vi "Auto Transmission and Manual control.vi"(0 "Drive":T4, 1 "Force which gear it is in":bool, 3 "Forced high gear?":bool, 5 "Commanded speeds":cluster{"Steer":dbl, "Throttle":dbl}, 9 "from Shift":T1, 11 "error in (no error)":errorcluster, 12 "All Shifter Constants":T2) -> (4 "Drive out":T4, 6 "in High Gear?":bool, 8 "Robot speed in FPS":dbl, 10 "To shift":T1, 14 "Recomended Gear (may be in that gear)":bool, 15 "error out":errorcluster)   [LabVIEW 2013]
uses:
  Drive typedef.ctl
  Drive Motors Typedef.ctl
  GearBox Typedef.ctl
  <vilib>/Rock Robotics/WPI/MotorControl/WPI_MotorControlDeviceRef.ctl
  <vilib>/Rock Robotics/SystemInterfaces/Typedef/FPGA_TypedefDigitalModule.ctl
  <vilib>/Rock Robotics/SystemInterfaces/DIO/FPGA_DIOPWMChannel.ctl
  <vilib>/Rock Robotics/WPI/PWM/WPI_PWMDeadband.ctl
  <vilib>/Rock Robotics/WPI/CAN/Jaguar/SubVIs/WPI_CANJaguar_ControlMode.ctl
  <vilib>/Rock Robotics/WPI/PWM/WPI_PWMTransform_ConPane.ctl
  <vilib>/Rock Robotics/WPI/Solenoid/WPI_SolenoidDevRef.ctl
  <vilib>/Rock Robotics/SystemInterfaces/Typedef/FPGA_TypedefSolenoidModule.ctl
  <vilib>/Rock Robotics/WPI/Solenoid/WPI_SolenoidChannel.ctl
  Drive Sensor Typedef.ctl
  <vilib>/Rock Robotics/WPI/Encoder/WPI_EncoderDevRef.ctl
  <vilib>/Rock Robotics/SystemInterfaces/Encoder/FPGA_EncoderIdx.ctl
  <vilib>/Rock Robotics/SystemInterfaces/Counter/FPGA_CounterCtrSystemIndex.ctl
  <vilib>/Rock Robotics/WPI/Encoder/WPI_EncoderType.ctl
  <vilib>/Rock Robotics/WPI/Gyro/WPI_GyroDevRef.ctl
  <vilib>/Rock Robotics/SystemInterfaces/Typedef/FPGA_TypedefAnalogModule.ctl
  <vilib>/Rock Robotics/SystemInterfaces/AI/FPGA_AIChannel.ctl
  All Shifter Constants.ctl
  Shift Constants.ctl
  Shifter shift typedef.ctl
  <vilib>/Rock Robotics/WPI/Solenoid/WPI_SolenoidValue.ctl
  <vilib>/Rock Robotics/WPI/Solenoid/Deprecated/WPI_SolenoidGetBool.vi
  <vilib>/Rock Robotics/WPI/Solenoid/WPI_SolenoidSetEnum.vi
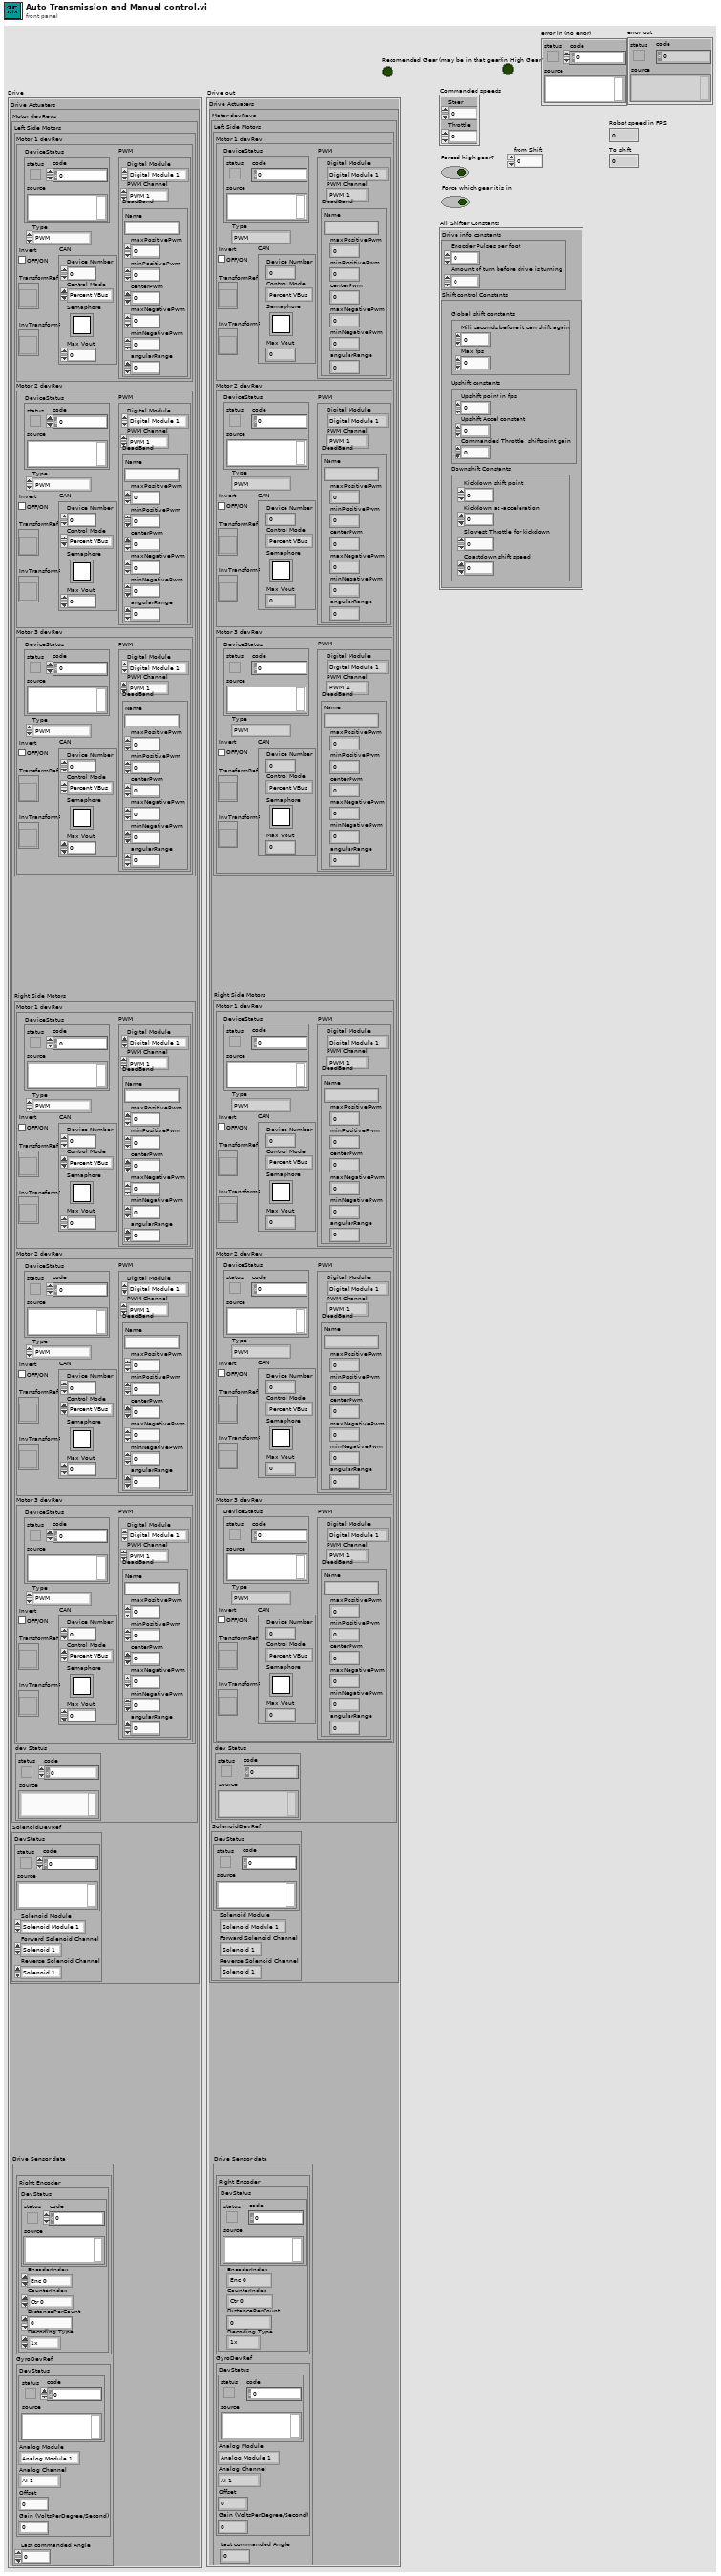
[diagram p1: front panel]
types:
  T1 = typedef "Shifter shift typedef.ctl" = u32
  T2 = typedef "All Shifter Constants.ctl" = cluster{"Drive info constants":cluster{"Enocder Pulses per foot":dbl, "Amount of turn before drive is turning":dbl}, "Shift control Constants":T3}
  T3 = typedef "Shift Constants.ctl" = cluster{"Global shift constants":cluster{"Mili seconds before it can shift again":u32, "Max fps":dbl}, "Upshift constants":cluster{"Upshift point in fps":dbl, "Upshift Accel constant":dbl, "Commanded Throttle  shiftpoint gain":dbl}, "Downshift Constants":cluster{"Kickdown shift point":dbl, "Kickdown at -acceleration":dbl, "Slowest Throttle for kickdown":dbl, "Coastdown shift speed":dbl}}
  T4 = typedef "Drive typedef.ctl" = cluster{"Drive Actuaters":cluster{"Motor devRevs":T5, "SolenoidDevRef":T14}, "Drive Sensor data":T17}
  T5 = typedef "Drive Motors Typedef.ctl" = cluster{"Left Side Motors":T6, "Right Side Motors":T6, "dev Status":errorcluster}
  T6 = typedef "GearBox Typedef.ctl" = cluster{"Motor 1 devRev":T7, "Motor 2 devRev":T7, "Motor 3 devRev":T7}
  T7 = typedef "WPI_MotorControlDeviceRef.ctl" = cluster{"DeviceStatus":errorcluster, "Type":enum16{"PWM", "CAN"}, "PWM":cluster{"Digital Module":T8, "PWM Channel":T9, "DeadBand":T10}, "CAN":cluster{"Device Number":u8, "Control Mode":T11, "Semaphore":T12, "Max Vout":dbl}, "Invert":bool, "TransformRef":T13, "InvTransformRef":T13}
  T8 = typedef "FPGA_TypedefDigitalModule.ctl" = enum16{"Digital Module 1", "Digital Module 2"}
  T9 = typedef "FPGA_DIOPWMChannel.ctl" = enum8{"PWM 1", "PWM 2", "PWM 3", "PWM 4", "PWM 5", "PWM 6", "PWM 7", "PWM 8", "PWM 9", "PWM 10", "Invalid"}
  T10 = typedef "WPI_PWMDeadband.ctl" = cluster{"Name":string, "maxPositivePwm":i32, "minPositivePwm":i32, "centerPwm":i32, "maxNegativePwm":i32, "minNegativePwm":i32, "angularRange":u16}
  T11 = typedef "WPI_CANJaguar_ControlMode.ctl" = enum8{"Percent VBus", "Current", "Speed", "Position", "Voltage"}
  T12 = typedef "Semaphore RefNum" = refnum<k1>
  T13 = typedef "WPI_PWMTransform_ConPane.ctl" = refnum<vi>
  T14 = typedef "WPI_SolenoidDevRef.ctl" = cluster{"DevStatus":errorcluster, "Solenoid Module":T15, "Forward Solenoid Channel":T16, "Reverse Solenoid Channel":T16}
  T15 = typedef "FPGA_TypedefSolenoidModule.ctl" = enum16{"Solenoid Module 1", "Solenoid Module 2"}
  T16 = typedef "WPI_SolenoidChannel.ctl" = enum8{"Solenoid 1", "Solenoid 2", "Solenoid 3", "Solenoid 4", "Solenoid 5", "Solenoid 6", "Solenoid 7", "Solenoid 8", "Invalid"}
  T17 = typedef "Drive Sensor Typedef.ctl" = cluster{"Encoders":cluster{"Right Encoder":T18}, "GyroDevRef":T22, "Last commanded Angle":dbl}
  T18 = typedef "WPI_EncoderDevRef.ctl" = cluster{"DevStatus":errorcluster, "EncoderIndex":T19, "CounterIndex":T20, "DistancePerCount":dbl, "Decoding Type":T21}
  T19 = typedef "FPGA_EncoderIdx.ctl" = enum8{"Enc 0", "Enc 1", "Enc 2", "Enc 3", "Invalid"}
  T20 = typedef "FPGA_CounterCtrSystemIndex.ctl" = enum8{"Ctr 0", "Ctr 1", "Ctr 2", "Ctr 3", "Ctr 4", "Ctr 5", "Ctr 6", "Ctr 7", "Invalid"}
  T21 = typedef "WPI_EncoderType.ctl" = enum16{"1x", "2x", "4x"}
  T22 = typedef "WPI_GyroDevRef.ctl" = cluster{"DevStatus":errorcluster, "Analog Module":T23, "Analog Channel":T24, "Offset":dbl, "Gain (VoltsPerDegree/Second)":dbl}
  T23 = typedef "FPGA_TypedefAnalogModule.ctl" = enum16{"Analog Module 1", "Analog Module 2"}
  T24 = typedef "FPGA_AIChannel.ctl" = enum8{"AI 1", "AI 2", "AI 3", "AI 4", "AI 5", "AI 6", "AI 7", "AI 8", "Invalid"}
  T25 = typedef "WPI_SolenoidValue.ctl" = enum16{"Off", "On", "Forward", "Reverse"}
  T26 = cluster{"Enocder Pulses per foot":dbl, "Amount of turn before drive is turning":dbl}
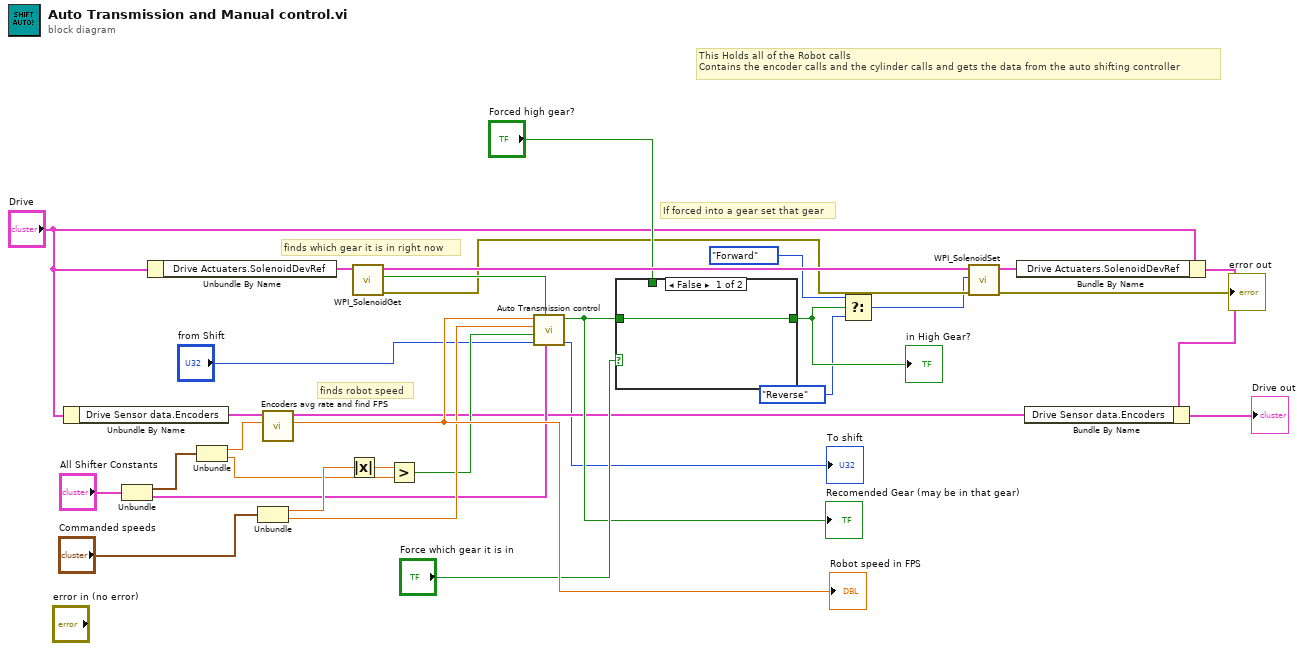
[diagram p0: block diagram]
diagram:
  # "finds which gear it is in right now"
  # "finds robot speed"
  # "If forced into a gear set that gear"
  # "This Holds all of the Robot calls\nContains the encoder calls and the cylinder calls and gets the data from the auto shifting controller"
  n1 = Unbundle By Name("Drive") -> ("Drive Sensor data.Encoders"=w31:cluster{"Right Encoder":T18})
  n2 = Unbundle("All Shifter Constants") -> ("Drive info constants"=w17:T26, "Shift control Constants"=w14:T3)
  n3 = Unbundle By Name("Drive") -> ("Drive Actuaters.SolenoidDevRef"=w29:T14)
  n4 = Unbundle(w17) -> ("Enocder Pulses per foot"=w16:dbl, "Amount of turn before drive is turning"=w15:dbl)
  n5 = Unbundle("Commanded speeds") -> ("Steer"=w25:dbl, "Throttle"=w26:dbl)
  n6 = call "Encoders avg rate and find FPS.vi"("encoder clicks per foot"=w16, "Encoders"=w31) -> ("Robot speed in FPS"=w30:dbl, "Encoders out"=w9:cluster{"Right Encoder":T18})  [unwired: 6 in, 2 out]
  "Robot speed in FPS" <- w30
  n7 = Absolute Value(x=w25) -> (abs(x)=w24:dbl)
  n8 = call-poly <vilib>:"WPI_SolenoidGet.vi"("SolenoidDevRef"=w29) -> ("error out"=w6:errorcluster, "Value"=w28:bool, "SolenoidDevRef"=w22:T14)  [unwired: 8 in]
  n9 = Greater?(x=w24, y=w15) -> (0:w23:bool)
  n10 = call "Auto Transmission control.vi"("Shift Constants"=w14, "In High Gear?"=w28, "Time of last recomended shift"="from Shift", "Is Turning?"=w23, "Commanded Throttle"=w26, "Avg  encoder speed in fps"=w30) -> ("Time of last recomended shift"=→"To shift":u32, "should be High Gear?"=w20:bool)  [unwired: 4 in]
  "Recomended Gear (may be in that gear)" <- w20
  n11 = case shown="False" "Force which gear it is in" {
    tunnel: w20 -> [w32 _]
    tunnel: "Forced high gear?" -> [_ w33]
    tunnel: [w32 w33] -> w4
    frame False {
    }
    frame True {
    }
  }
  "in High Gear?" <- w4
  n12 = Select(t=WPI_SolenoidValue."Forward" ("Value"), s=w4, f=WPI_SolenoidValue."Reverse" ("Value")) -> (s? t:f=w1:T25)
  n13 = call-poly <vilib>:"WPI_SolenoidSet.vi"("error in (no error)"=w6, "Value"=w1, "SolenoidDevRef"=w22) -> ("error out"=→"error out":errorcluster, "SolenoidDevRef"=w12:T14)  [unwired: 7 in]
  n14 = Bundle By Name(cluster="Drive", "Drive Actuaters.SolenoidDevRef"=w12) -> (w11:T4)
  n15 = Bundle By Name(cluster=w11, "Drive Sensor data.Encoders"=w9) -> (→"Drive out":T4)
